vi "EnsureUnique.vi"(2 "Existing Targets Hit":string[](array[string]), 3 "Potentially New Targets Hit":string[](array[string])) -> (0 "Existing Targets Hit Updated":string[](array[string]), 1 "New Targets Hit":string[](array[string]))   [LabVIEW 2015, in "Level.lvclass"]
uses:
  Level.lvclass
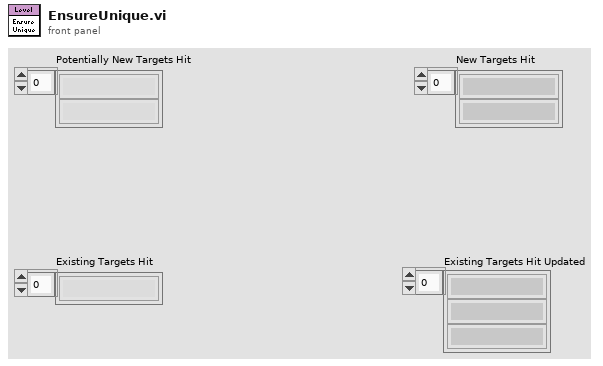
[diagram p1: front panel]
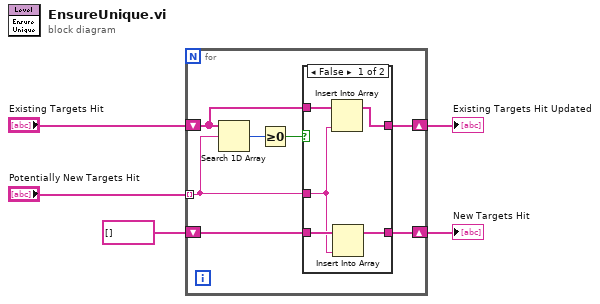
[diagram p0: block diagram]
diagram:
  n1 = for {
    tunnel: "Potentially New Targets Hit" -> [w9] mode=indexing
    shift-right: [w8] -> w2
    shift-left: string[] [] ("Potentially New Targets Hit 2") -> [w10]
    shift-right: [w6] -> w1
    shift-left: "Existing Targets Hit" -> [w7]
    n2 = Search 1D Array(1D array=w7, element=w9) -> (index of element=w12:i32)  [unwired: 1 in]
    n3 = Greater Or Equal To 0?(x=w12) -> (x >= 0?=w11:bool)
    n4 = case shown="False" w11 {
      tunnel: w10 -> [w17 w19]
      tunnel: w9 -> [w13 _]
      tunnel: [w16 w19] -> w8
      tunnel: w7 -> [w15 w18]
      tunnel: [w14 w18] -> w6
      frame False {
        n5 = Insert Into Array(array=w15, new element=w13) -> (w14:string[])  [unwired: 1 in]
        n6 = Insert Into Array(array=w17, new element=w13) -> (w16:string[])  [unwired: 1 in]
      }
      frame True {
      }
    }
  }
  "New Targets Hit" <- w2
  "Existing Targets Hit Updated" <- w1
